vi "Tektronix DPO MSO 2000 4000 Series Configure and Read Frequency Domain Measurements.vi"() -> ()   [LabVIEW 2010]
doc: "This example illustrates how to configure and read a Frequency Domain Measurement for the MDO series oscilloscopes.\n\n<B>Note:</B>\n This example is applicable only to <B>MDO series</B> oscilloscopes."
uses:
  <instrlib>/Tektronix DPO MSO 2000 4000 Series/Tektronix DPO MSO 2000 4000 Series.lvlib
panel:
  out "Units":u16(ring) items=["dBm", "dBµW", "dBmV", "dbµV", "dbmA", "dBµA"]
  out "Channel Power":dbl
  in  "Percentage of Power (60%)":dbl=60.0 min=60.0 max=99.9 step=0.1 format="%#_g %"
  in  "Spacing Units (0:Hz)":u16(ring) items=["Hz", "kHz", "MHz", "GHz"]
  in  "Channel Spacing (14)":dbl=14.0 min=14.0
  in  "Number of Adjacent Channels (1)":i8=1 min=1 max=3 step=1
  in  "Units (0:Hz)":u16(ring) items=["Hz", "KHz", "MHz", "GHz"]
  in  "Channel BandWidth (0)":dbl
  in  "Measurement (0:None)":u16(ring) items=["None", "Channel Power", "Adjacent Channel Power Ratio", "Occupied Bandwidth"]
  in  "VISA Resource Name":refnum<visa-resource-name>
  # "(c) 2006 - 2012. National Instruments Corporation. ALL RIGHTS RESERVED."
  # "All Measurements"
  # "Measurement Result"
  # "Adjacent Channel Power Ratio Measurement"
  # "Occupied Bandwidth Measurement"
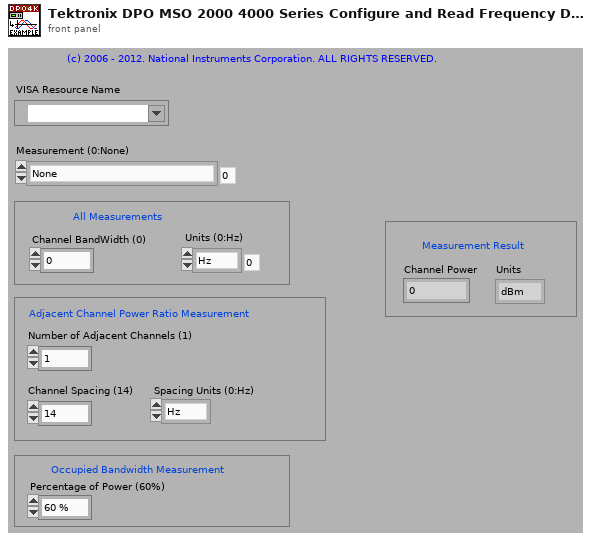
[diagram p1: front panel]
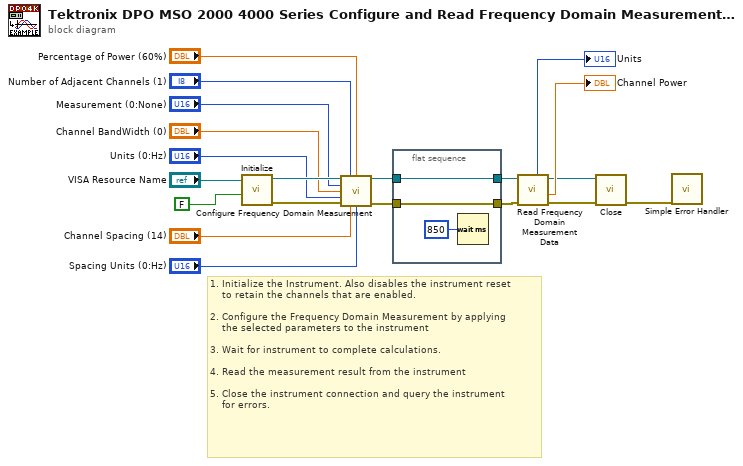
[diagram p0: block diagram]
diagram:
  # "1. Initialize the Instrument. Also disables the instrument reset\n    to retain the channels that are enabled.\n\n2. Configure the Frequency Domain Measurement by applying\n    the selected parameters to the instrument\n\n3. Wait for instrument to complete calculations.\n\n4. Read the measurement result from the instrument\n\n5. Close the instrument connection and query the instrument\n    for errors."
  n1 = call <instrlib>:"Initialize.vi"("Reset (True)"=FALSE, "VISA resource name"="VISA Resource Name") -> ("error out"=w17:errorcluster, "VISA resource name out"=w18:refnum<visa-resource-name>)  [unwired: 8 in]
  n2 = call <instrlib>:"Configure Frequency Domain Measurement.vi"("VISA resource name"=w18, "Number of Adjacent Channels (1)"="Number of Adjacent Channels (1)", "Percentage of Power (60%)"="Percentage of Power (60%)", "Measurement (0:None)"="Measurement (0:None)", "Channel BandWidth (0)"="Channel BandWidth (0)", "Units (0:Hz)"="Units (0:Hz)", "error in (no error)"=w17, "Channel Spacing (14 Hz)"="Channel Spacing (14)", "Spacing Units (0:Hz)"="Spacing Units (0:Hz)") -> ("VISA resource name out"=w4:refnum<visa-resource-name>, "error out"=w3:errorcluster)  [unwired: 5 in]
  n3 = flat-sequence {
    tunnel: w4 -> [w23]
    tunnel: w3 -> [w22]
    tunnel: [w23] -> w2
    tunnel: [w22] -> w1
    frame #0 {
      n4 = Wait (ms)(milliseconds to wait=u32 850) -> ()  [unwired: 1 out]
    }
  }
  n5 = call <instrlib>:"Read Frequency Domain Measurement Data.vi"("error in (no error)"=w1, "VISA resource name"=w2) -> ("error out"=w6:errorcluster, "Channel Power"=→"Channel Power":dbl, "VISA resource name out"=w7:refnum<visa-resource-name>, "Units"=→"Units":u16)  [unwired: 5 in, 1 out]
  n6 = call <instrlib>:"Close.vi"("error in (no error)"=w6, "VISA resource name"=w7) -> ("error out"=w5:errorcluster)  [unwired: 9 in]
  n7 = call <vilib>:"Simple Error Handler.vi"("error in (no error)"=w5) -> ()  [unwired: 4 in, 5 out]
